vi "PM100D_set_fetch.vi"(8 "error in":errorcluster, 9 "Timeout [ms]":i32=1000, 10 "Averaging Rate":i32=300, 11 "VISA in":refnum<visa-resource-name>="COM1") -> (0 "error out":errorcluster, 1 "Readout value":dbl format="%^#_9e", 2 "Readout string":string, 3 "VISA out":refnum<visa-resource-name>, 5 "New":bool)   [LabVIEW 2014]
panel:
  out "Error log":string
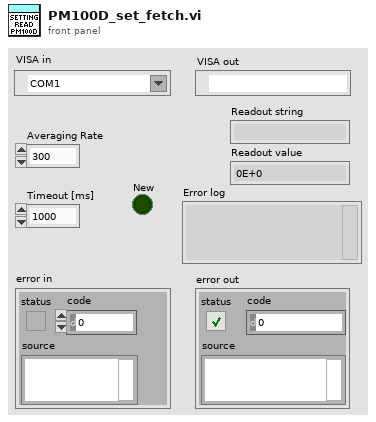
[diagram p1: front panel]
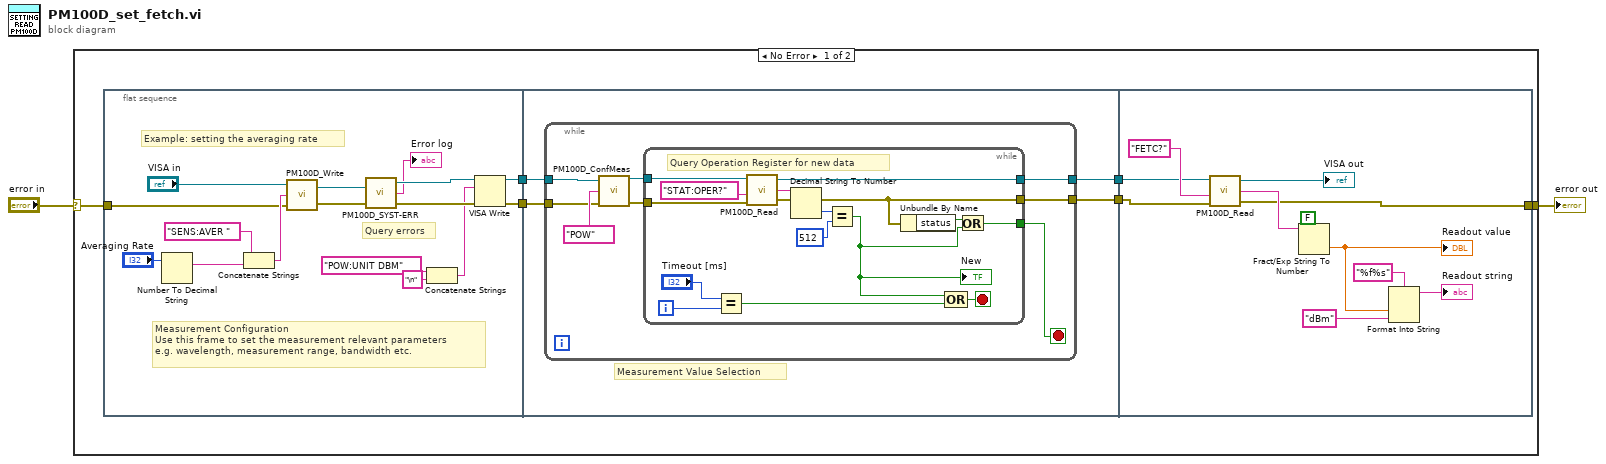
[diagram p0: block diagram]
diagram:
  n1 = case shown="No Error" "error in" {
    selector: "error in" -> [w4 w63]
    tunnel: [w3 w63] -> w2
    frame No Error {
      n2 = flat-sequence {
        tunnel: [w11] -> w8
        tunnel: [w10] -> w7
        tunnel: w4 -> [w9]
        tunnel: w8 -> [w28]
        tunnel: w7 -> [w27]
        tunnel: [w26] -> w6
        tunnel: [w25] -> w5
        tunnel: w6 -> [w55]
        tunnel: w5 -> [w54]
        tunnel: [w52] -> w3
        frame #0 {
          # "Query errors"
          # "Example: setting the averaging rate"
          # "Measurement Configuration\nUse this frame to set the measurement relevant parameters\ne.g. wavelength, measurement range, bandwidth etc."
          n3 = Number To Decimal String(number="Averaging Rate") -> (decimal integer string=w15:string)  [unwired: 1 in]
          n4 = Concatenate Strings("SENS:AVER " ("string"), w15) -> (w17:string)
          n5 = call "PM100D_Write.vi"("error in (no error)"=w9, "Command"=w17, "VISA in"="VISA in") -> ("error out"=w20:errorcluster, "VISA out"=w18:refnum<visa-resource-name>)
          n6 = call "PM100D_SYST-ERR.vi"("error out 2"=w20, "VISA In"=w18) -> ("error out"=w23:errorcluster, "Error"=→"Error log":string, "VISA Out"=w22:refnum<visa-resource-name>)  [unwired: 1 in]
          n7 = Concatenate Strings("POW:UNIT DBM" ("string"), "\n" ("String")) -> (w21:string)
          n8 = VISA Write(VISA resource name=w22, write buffer=w21, error in (no error)=w23) -> (VISA resource name out=w11:refnum<visa-resource-name>, error out=w10:errorcluster)  [unwired: 1 out]
        }
        frame #1 {
          # "Measurement Value Selection"
          n9 = while {
            tunnel: w27 -> [w32]
            tunnel: w28 -> [w31]
            tunnel: [w30] -> w25
            tunnel: [w29] -> w26
            stop <- w33 stop-if-true
            n10 = call "PM100D_ConfMeas.vi"("error in"=w32, "Conf:"="POW" ("Readout Config"), "VISA In"=w31) -> ("error out"=w35:errorcluster, "dup VISA session"=w36:refnum<visa-resource-name>)
            n11 = while {
              tunnel: w36 -> [w47]
              tunnel: w35 -> [w46]
              tunnel: [w45] -> w30
              tunnel: [w40] -> w29
              tunnel: [w37] -> w33
              i -> [w42]
              stop <- w44 stop-if-true
              # "Query Operation Register for new data"
              n12 = Equal?(x="Timeout [ms]", y=w42) -> (x = y?=w41:bool)
              n13 = call "PM100D_Read.vi"("error in (no error)"=w46, "Command"="STAT:OPER?", "VISA in"=w47) -> ("error out"=w40:errorcluster, "ReadValue"=w50:string, "VISA out"=w45:refnum<visa-resource-name>)  [unwired: 1 in]
              n14 = Decimal String To Number(string=w50) -> (number=w49:i32)  [unwired: 2 in, 1 out]
              n15 = Equal?(x=w49, y=512) -> (x = y?=w38:bool)
              "New" <- w38
              n16 = Unbundle By Name(w40) -> ("status"=w39:bool)
              n17 = Compound Arithmetic op=OR(w38, w41) -> (w44:bool)
              n18 = Or(x=w39, y=w38) -> (x .or. y?=w37:bool)
            }
          }
        }
        frame #2 {
          n19 = call "PM100D_Read.vi"("error in (no error)"=w55, "Command"="FETC?", "VISA in"=w54) -> ("error out"=w52:errorcluster, "ReadValue"=w61:string, "VISA out"=→"VISA out":refnum<visa-resource-name>)  [unwired: 1 in]
          n20 = Fract/Exp String To Number(use system decimal point (T)=FALSE, string=w61) -> (number=w58:dbl)  [unwired: 2 in, 1 out]
          "Readout value" <- w58
          n21 = Format Into String(format string="%f%s", w58, "dBm") -> (resulting string=→"Readout string":string)  [unwired: 2 in, 1 out]
        }
      }
    }
    frame Error {
    }
  }
  "error out" <- w2
